vi "CSTK_MCListbox_Designer_ModiifyColHdrsWidthBatches.vi"(8 "错误输入（无错误）":errorcluster, 9 "Width":u32, 10 "MulticolumnListbox输入":refnum<vi>, 11 "VI输入":refnum<vi>) -> (0 "错误输出":errorcluster, 3 "VI输出":refnum<vi>)   [LabVIEW 2015, in "CSTK_MCListbox Designer.lvlib"]
uses:
  CSTK_MCListbox Designer.lvlib
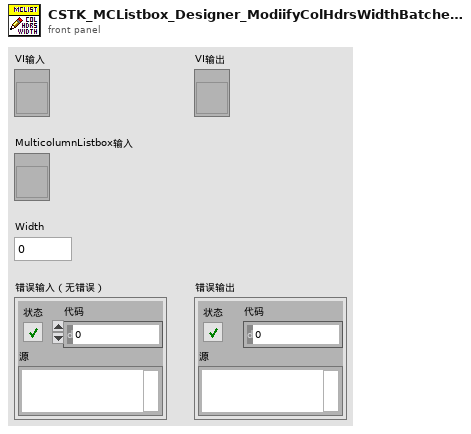
[diagram p1: front panel]
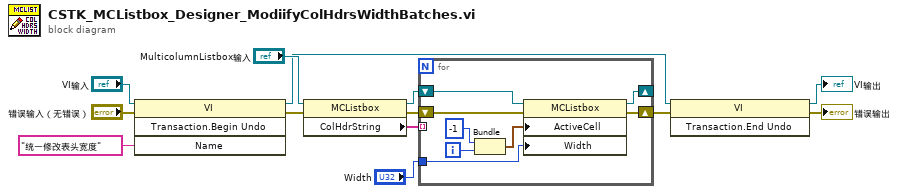
[diagram p0: block diagram]
diagram:
  n1 = invoke class="VI" method="Transaction.Begin Undo"(reference="VI输入", error in="错误输入（无错误）", "Name"="统一修改表头宽度" ("名称")) -> (reference out=w2:refnum<vi>, error out=w8:errorcluster)  [unwired: 1 in, 2 out]
  n2 = property class="MCListbox"(reference="MulticolumnListbox输入", error in=w8) -> (reference out=w11:refnum<vi>, error out=w9:errorcluster, "ColHdrString"=w12:string[])
  n3 = for {
    shift-right: [w17] -> _
    shift-left: w11 -> [w18]
    shift-right: [w15] -> w5
    shift-left: w9 -> [w16]
    tunnel: "Width" -> [w14]
    tunnel: w12 -> [_] mode=indexing
    i -> [w20]
    n4 = Bundle(-1, w20) -> (w19:cluster{i32, i32})  [unwired: 1 in]
    n5 = property class="MCListbox"(reference=w18, error in=w16, "ActiveCell"=w19, "Width"=w14) -> (reference out=w17:refnum<vi>, error out=w15:errorcluster)
  }
  n6 = invoke class="VI" method="Transaction.End Undo"(reference=w2, error in=w5) -> (reference out=→"VI输出":refnum<vi>, error out=→"错误输出":errorcluster)  [unwired: 1 in, 1 out]
